vi "createFolder.vi"() -> ()   [LabVIEW 2016]
panel:
  out "actual path":path
  out "file or folder exists?":bool
  in  "Pick a new filename":bool
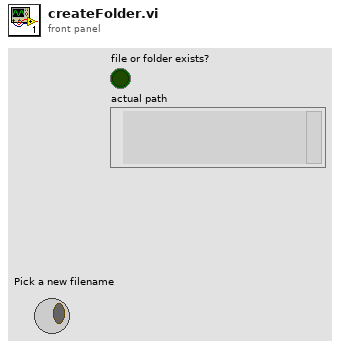
[diagram p1: front panel]
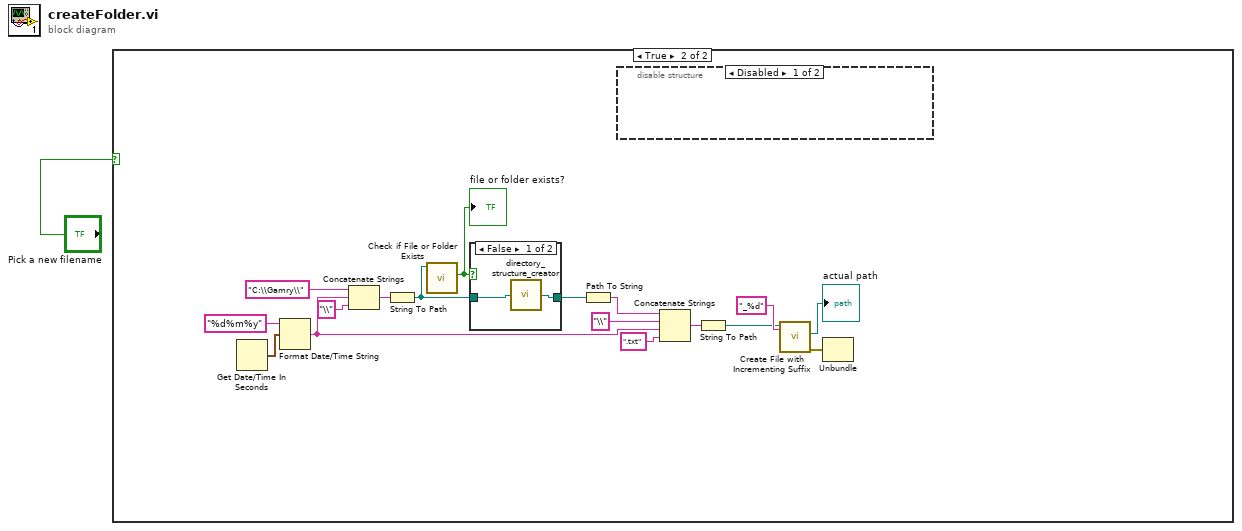
[diagram p0: block diagram]
diagram:
  n1 = case shown="True" "Pick a new filename" {
    frame False {
    }
    frame True {
      n2 = Get Date/Time In Seconds() -> (seconds since 1Jan1904=w13:timestamp)
      n3 = Format Date/Time String(time format string (%c)="%d%m%y" ("pattern"), seconds (now)=w13) -> (date/time string=w4:string)  [unwired: 1 in]
      n4 = Concatenate Strings("C:\\Gamry\\" ("default data"), w4, "\\" ("pattern")) -> (w2:string)
      n5 = String To Path(string=w2) -> (path=w15:path)
      n6 = call <vilib>:"Check if File or Folder Exists.vi"("path"=w15) -> ("file or folder exists?"=w16:bool)  [unwired: 8 in, 2 out]
      "file or folder exists?" <- w16
      n7 = case shown="False" w16 {
        tunnel: w15 -> [w20 w21]
        tunnel: [w19 w21] -> w14
        frame False {
          n8 = call "directory_structure_creator.vi"("Path to be created"=w20) -> ("Duplicate \"Path to be created\""=w19:path)
        }
        frame True {
        }
      }
      n9 = Path To String(path=w14) -> (string=w8:string)
      n10 = disable-structure shown="Disabled" {
        frame Disabled {
        }
        frame Enabled {
        }
      }
      n11 = Concatenate Strings(w8, "\\" ("pattern"), w4, ".txt" ("pattern")) -> (w6:string)
      n12 = String To Path(string=w6) -> (path=w10:path)
      n13 = call <vilib>:"Create File with Incrementing Suffix.vi"("format string (\" (%d)\")"="_%d" ("pattern"), "file path"=w10) -> ("error out"=w18:errorcluster, "actual path"=→"actual path":path)  [unwired: 7 in, 1 out]
      n14 = Unbundle(w18) -> ()  [unwired: 3 out]
    }
  }
